vi "Incrementer.vi"(1 "N":u64, 5 "error in (no error)":errorcluster caption="Fehler (Eingang, kein Fehler)") -> (6 "error out":errorcluster caption="Fehler (Ausgang)")   [LabVIEW 2016]
uses:
  File Progress Global.vi
panel:
  out "String":string
  out "Progress [%]":u64(slide) scale=0.0..100.0
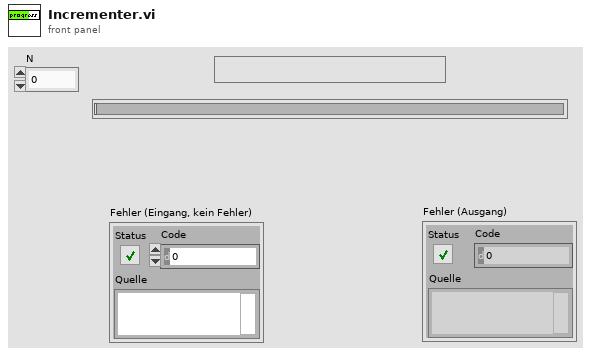
[diagram p1: front panel]
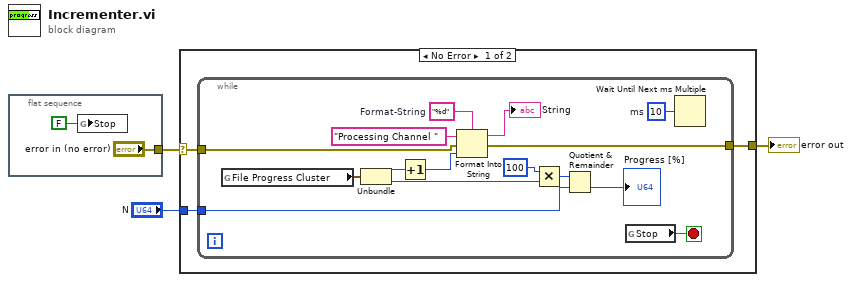
[diagram p0: block diagram]
diagram:
  n1 = flat-sequence {
    tunnel: ["error in (no error)"] -> w2
    frame #0 {
      n2 = global write "File Progress Global.vi" "Stop"(FALSE ("Stop")) -> ()
    }
  }
  n3 = case shown="No Error" w2 {
    selector: w2 -> [w8 w24]
    tunnel: [w7 w24] -> w3
    tunnel: "N" -> [w6 _]
    frame No Error {
      n4 = while {
        tunnel: w8 -> [w13]
        tunnel: [w12] -> w7
        tunnel: w6 -> [w9]
        stop <- w19 stop-if-true
        w16 = "%d"  # Format-String
        w18 = u32 10  # ms
        n5 = global read "File Progress Global.vi" "File Progress Cluster"() -> (w20:cluster{"Channel Count":i32, "Offset Count":i64})
        n6 = Unbundle(w20) -> ("Channel Count"=w11:i32, "Offset Count"=w14:i64)
        n7 = Increment(x=w11) -> (x+1=w10:i32)
        n8 = Format Into String(format string=w16, initial string="Processing Channel ", error in=w13, w10) -> (resulting string=→"String":string, error out=w12:errorcluster)
        n9 = Multiply(x=u64 100, y=w14) -> (x*y=w23:u64)
        n10 = Quotient & Remainder(x=w23, y=w9) -> (floor(x/y)=→"Progress [%]":u64)  [unwired: 1 out]
        n11 = global read "File Progress Global.vi" "Stop"() -> (w19:bool)
        n12 = Wait Until Next ms Multiple(millisecond multiple=w18) -> ()  [unwired: 1 out]
      }
    }
    frame Error {
    }
  }
  "error out" <- w3
